vi "TriggerScopeCollect.vi"(8 "error in (no error)":errorcluster, 10 "period":dbl=1.0 min=0.0001 max=8.0 step=1.0, 11 "controller in":refnum<k24>) -> (0 "error out":errorcluster, 3 "controller out":refnum<k24>)   [LabVIEW 2019]
uses:
  C:/Users/patrick/Documents/GitHub/Aerotech-Delay-Line/lvsrc/Aerotech-Ensemble-LabVIEW/2010-5.6/Bin/Aerotech.Ensemble.dll
  Bin/Aerotech.Ensemble.dll
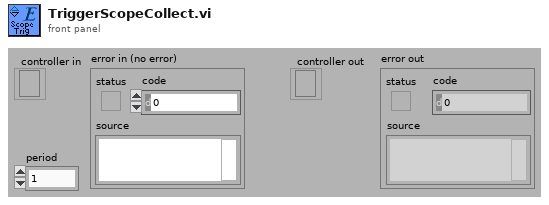
[diagram p1: front panel]
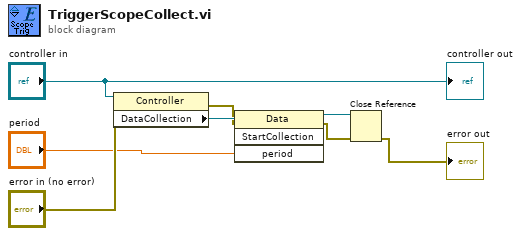
[diagram p0: block diagram]
diagram:
  n1 = property class="Controller"(reference="controller in", error in="error in (no error)") -> (error out=w5:errorcluster, "DataCollection"=w6:refnum<k24>)  [unwired: 1 out]
  n2 = invoke class="Data" method="StartCollection"(reference=w6, error in=w5, "period"="period") -> (reference out=w1:refnum<k24>, error out=w3:errorcluster)  [unwired: 1 in, 2 out]
  n3 = Close Reference(reference=w1, error in (no error)=w3) -> (error out=→"error out":errorcluster)
  "controller out" <- "controller in"
